vi "S2C_CMD_TranslateSettings.vi"(8 "Error In":errorcluster, 11 "Data":variant) -> (0 "Error Out":errorcluster, 3 "JSON Cluster":string)   [LabVIEW 2015]
doc: "Translates a JSON flattened 2D array into a flattened JSON cluster. The cluster can then be accessed by parameter name. Used specifically to access the step setting parameters."
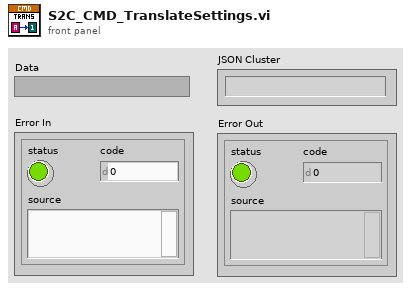
[diagram p1: front panel]
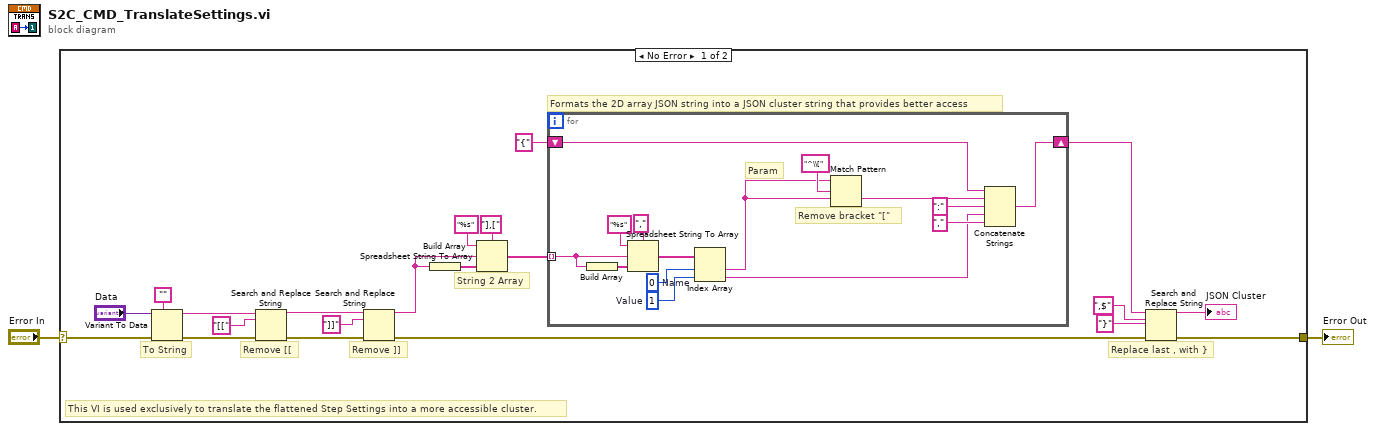
[diagram p0: block diagram]
diagram:
  n1 = case shown="No Error" "Error In" {
    selector: "Error In" -> [w6 w37]
    tunnel: [w11 w37] -> w1
    frame No Error {
      # "This VI is used exclusively to translate the flattened Step Settings into a more accessible cluster."
      # "To String"
      # "Remove ]]"
      # "Formats the 2D array JSON string into a JSON cluster string that provides better access"
      # "Replace last , with }"
      # "String 2 Array"
      # "Remove [["
      n2 = Variant To Data(error in=w6, type="", Variant="Data") -> (data=w3:string, error out=w5:errorcluster)
      n3 = Search and Replace String(input string=w3, search string="[[", error in=w5) -> (result string=w9:string, error out=w12:errorcluster)  [unwired: 5 in, 2 out]
      n4 = Search and Replace String(input string=w9, search string="]]") -> (result string=w8:string)  [unwired: 6 in, 3 out]
      n5 = Build Array(w8) -> (w19:string[])
      n6 = Spreadsheet String To Array(delimiter (Tab)="],[", format string="%s", spreadsheet string=w8, array type (2D Dbl)=w19) -> (array=w18:string[])
      n7 = for {
        tunnel: w18 -> [w25] mode=indexing
        shift-right: [w33] -> w17
        shift-left: "{" -> [w34]
        w26 = 1  # Value
        w27 = 0  # Name
        # "Remove bracket \"[\""
        # "Param"
        n8 = Build Array(w25) -> (w29:string[])
        n9 = Spreadsheet String To Array(delimiter (Tab)=",", format string="%s", spreadsheet string=w25, array type (2D Dbl)=w29) -> (array=w28:string[])
        n10 = Index Array(array=w28, index #1=w27, index #2=w26) -> (element #1=w24:string, element #2=w23:string)
        n11 = Match Pattern(string=w24, regular expression="^\\[") -> ()  [unwired: 1 in, 4 out]
        n12 = Concatenate Strings(w34, w24, ":" ("string"), w23, "," ("string")) -> (w33:string)
      }
      n13 = Search and Replace String(input string=w17, search string=",$", replace string="}" ("replace string (\"\")"), error in=w12) -> (result string=→"JSON Cluster":string, error out=w11:errorcluster)  [unwired: 4 in, 2 out]
    }
    frame Error {
    }
  }
  "Error Out" <- w1
